vi "Calculate Y Parameters (SubVI).vi"(10 "Camera":i32[][](array[numeric]), 11 "DMD":i32[][](array[numeric])) -> (3 "Polynomial Coefficients":dbl[](array[numeric]))   [LabVIEW 2017]
uses:
  <vilib>/Analysis/NI_AALPro.lvlib
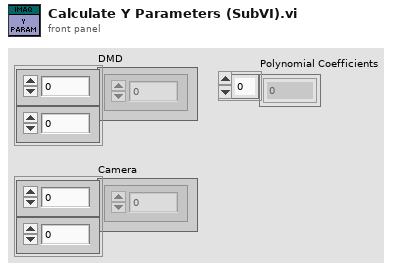
[diagram p1: front panel]
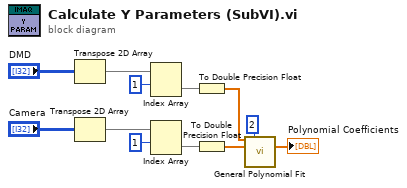
[diagram p0: block diagram]
diagram:
  n1 = Transpose 2D Array(2D array="DMD") -> (transposed array=w6:i32[][])
  n2 = Transpose 2D Array(2D array="Camera") -> (transposed array=w9:i32[][])
  n3 = Index Array(array=w6, index (row)=1) -> (element=w5:i32[])  [unwired: 1 in]
  n4 = Index Array(array=w9, index (row)=1) -> (element=w11:i32[])  [unwired: 1 in]
  n5 = To Double Precision Float(number=w5) -> (double precision float=w3:dbl[])
  n6 = To Double Precision Float(number=w11) -> (double precision float=w10:dbl[])
  n7 = call <vilib>:"General Polynomial Fit.vi"("Y"=w3, "polynomial order"=2, "X"=w10) -> ("Polynomial Coefficients"=→"Polynomial Coefficients":dbl[])  [unwired: 9 in, 3 out]
